vi "fgv_load-param.vi"(7 "cmd":T2, 8 "error in":errorcluster caption="error", 11 "TestType":T1=enum."Reg") -> (0 "error out":errorcluster caption="eror out")   [LabVIEW 2019]
uses:
  load-save_param.ctl
  _ctrl/TestType.ctl
  _ctrl/rw.ctl
  Global_params.vi
  Register/Global_params_reg.vi
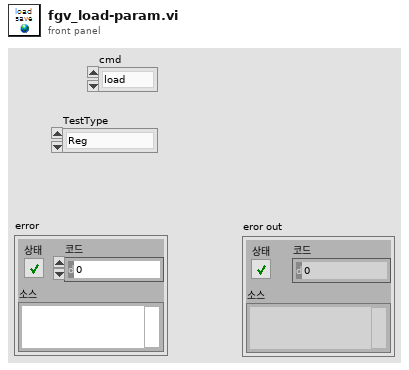
[diagram p1: front panel]
types:
  T1 = typedef "TestType.ctl" = enum16{"Manual", "Reg", "Cap", "B1", "B2", "B3"}
  T2 = typedef "load-save_param.ctl" = enum16{"load", "save"}
  T3 = typedef "rw.ctl" = enum16{"read", "write"}
  T4 = typedef "config_aging.ctl" = cluster{"Setting":T5, "TestName":string, "Result path":path, "파일 생성 주기[N]":u8, "Test Specs":T6}
  T5 = typedef "Setting_reg.ctl" = cluster{"제어 전압[V]":dbl, "출력전압[V]":dbl, "전류[A]":dbl, "출력전류[A]":dbl, "ON[초]":dbl, "OFF[초]":dbl, "Irms 허용치 from ":dbl, "Irms 허용치 to":dbl, "AO Delay ms":u32, "Log":path, "result":path}
  T6 = typedef "Breakdown-Spec.ctl" = cluster{"제어단 단선 Irms[mA](이하)":dbl, "제어단 특성 전류 Irms[mA] Max":dbl, "제어단 특성 전류 Irms[mA] Min":dbl, "출력단 단선 Irms[mA](이하)":dbl, "출력단 특성 전류 Irms[mA]  Max":dbl, "출력단 특성전류 Irms[mA]  Min":dbl, "온도[degree]":dbl}
  T7 = typedef "DL950_config.ctl" = cluster{"Timeout":u32, "Time Div":i32, "Acq Mode":i32, "Record Len":i32, "Record Num":i32, "Start Point":i64, "End Poin":i64, "Visa":refnum<visa-resource-name>, "Config Voltage":cluster{"Enable":bool, "Ch":u16, "V Div":i32, "Coupling":i32, "Probe":i32, "Act.Items":bool, "items":i32[]}[], "Trigger on":bool, "Trigger Level":dbl, "Reset":bool, "Config Temp":cluster{"Channel":u16, "Burn Out":bool, " Type ":i32}[], "Trig Mode":i32, "Trig Pos":dbl, "Trigger Slope":i32, "Trigger Source ":i32, "Trig Start -5":dbl, "End 5":dbl}
  T8 = typedef "BP4610_config.ctl" = cluster{"VISA":refnum<visa-resource-name>, "Limit-BP":cluster{"Set":enum16{"Current", "Voltage"}, "Voltage+[V]":dbl, "Current+[A]":dbl, "Voltage-[V]":dbl, "Current-[A]":dbl}, "SET BP":cluster{"Set":enum16{"Current", "Voltage", "FREQ/WAVE"}, "Operation mode":u16, "Voltage[Vp-p]":dbl, "Current[Ap-p]":dbl, "Voltage[V]":dbl, "Current[A]":dbl, "Frequency[Hz]":dbl, "Waveform":enum16{"Sine", "Square", "ARB 1", "ARB 2", "ARB 3", "ARB 4", "ARB 5", "ARB 6", "ARB 7", "ARB 8", "ARB 9", "ARB 10", "ARB 11", "ARB 12", "ARB 13", "ARB 14", "ARB 15", "ARB 16"}}}
  T9 = typedef "DSP_config.ctl" = cluster{"Port":refnum<visa-resource-name>, "OVP Level":dbl, "OCP Level":dbl, "Current":dbl, "Voltage":dbl}
  T10 = typedef "Set_NIAI.ctl" = cluster{"input terminal":i32, "minimum value":dbl, "maximum value":dbl, "number of samples":i32, "rate":dbl, "sample mode":i32, "physical channels":tag}
  T11 = typedef "cDAQ-9269 Config.ctl" = cluster{"Ch":tag, "Max V":dbl, "Min V":dbl, " Rate":dbl, "N pts":i32, "sample mode":i32}
  T12 = typedef "Set_AO_Wave-config.ctl" = cluster{"offset":dbl, "Samples":i32, "duty":dbl, "Rate":dbl, "wfm":cluster{"Freq":dbl, "Amp":dbl, "Type":enum16{"Sine Wave", "Triangle Wave", "Square Wave", "Sawtooth Wave"}}}
  T13 = cluster{"Params":T4, "DL950_config":T7, "BP4610 Config":T8, "DSP1950 Config":T9, "DMM 2470 Config":cluster{"Source Mode":enum16{"Voltage", "Current"}, "Source Limit Level":dbl, "Source Level":dbl, "Output_2470":bool}, "cDAQ-9221 Config":T10, "cDAQ-9467 Config":tag, "cDAQ-9269 AO Config":T11, "AO_Wave-config":T12}
  T14 = typedef "Testing-info.ctl" = cluster{"전체채널수":u8, "현재채널번호":u8, "Irms":dbl, "입력전압":dbl, "입력전류":dbl, "출력전압":dbl, "출력전류":dbl, "온도":dbl, "제어단 단선":bool, "제어단 단락":bool, "제어단 특성변화":bool, "출력단 단선":bool, "출력단 단락":bool, "출력단 특성변화":bool, "출력단 전압":bool, "카운트 일치":bool, "Irms 판정":bool, "온도":bool, "테스트 회수":u32, "TestType":T15, "현재회수":u32, "Ch selection":cluster{"1ch":bool, "2ch":bool, "3ch":bool, "4ch":bool, "5ch":bool, "6ch":bool}, "반복":u32, "Path":path, "파일생성주기":u32, "start time":dbl, "stop time":dbl, "현재반복회수":u32, "NG":cluster{"입출력 카운트":bool, "출력전류RMS":bool}}
  T15 = typedef "sequence_single.ctl" = enum16{"Register", "RC", "B1", "B2", "B3"}
  T16 = cluster{"DL950_config":T7, "BP4610 Config":T8, "DSP1950 Config":T9, "DMM 2470 Config":cluster{"Source Mode":enum16{"Voltage", "Current"}, "Source Limit Level":dbl, "Source Level":dbl, "Output_2470":bool}, "cDAQ-9221 Config":T10, "cDAQ-9467 Config":tag, "cDAQ-9269 AO Config":T11, "AO_Wave-config":T12}
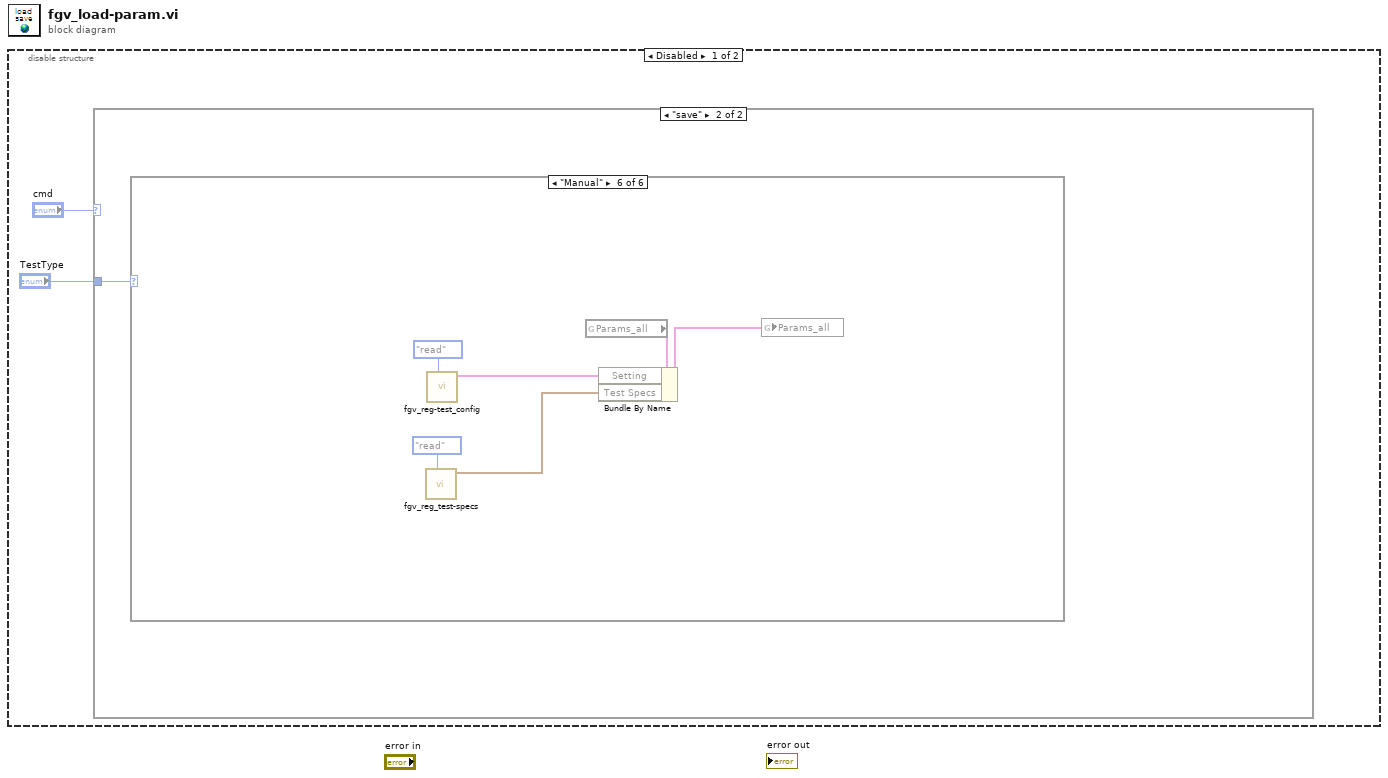
[diagram p0: block diagram]
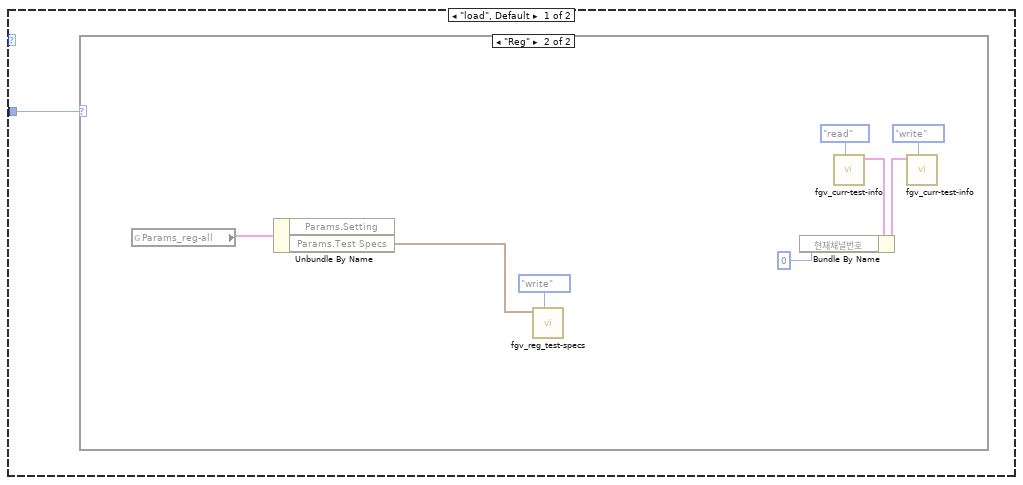
[diagram p2: hidden frame]
diagram:
  n1 = disable-structure shown="Disabled" {
    frame Disabled {
      n2 = case shown="\"save\"" "cmd" {
        tunnel: "TestType" -> [w3 w12]
        frame "load", Default {
          n3 = case shown="\"Reg\"" w3 {
            frame "Manual", Default {
            }
            frame "Reg" {
              n4 = global read "Global_params_reg.vi" "Params_reg-all"() -> (w4:T13)
              n5 = Unbundle By Name(w4) -> ("Params.Test Specs"=w6:T6)  [unwired: 1 out]
              n6 = call "fgv_reg_test-specs.vi"("cmd"=rw."write", "고장진단 기준 값"=w6) -> ()  [unwired: 9 in, 1 out]
              n7 = call "fgv_curr-test-info.vi"("cmd"=rw."read") -> ("현재테스트 정보 2"=w9:T14)  [unwired: 10 in]
              n8 = Bundle By Name(cluster=w9, "현재채널번호"=u8 0) -> (w8:T14)
              n9 = call "fgv_curr-test-info.vi"("cmd"=rw."write", "현재테스트 정보"=w8) -> ()  [unwired: 9 in, 1 out]
            }
          }
        }
        frame "save" {
          n10 = case shown="\"Manual\"" w12 {
            frame "Reg", Default {
            }
            frame "Cap" {
            }
            frame "B1" {
            }
            frame "B2" {
            }
            frame "B3" {
            }
            frame "Manual" {
              n11 = call "fgv_reg_test-specs.vi"("cmd"=rw."read") -> ("고장진단 기준 값 2"=w15:T6)  [unwired: 10 in]
              n12 = call "fgv_reg-test_config.vi"("cmd"=rw."read") -> ("TestConfig out"=w17:T5)  [unwired: 10 in]
              n13 = global read "Global_params.vi" "Params_all"() -> (w14:T16)
              n14 = Bundle By Name(cluster=w14, "Setting"=w17, "Test Specs"=w15) -> (w13:T16)
              n15 = global write "Global_params.vi" "Params_all"(w13) -> ()
            }
          }
        }
      }
    }
    frame Enabled {
    }
  }
